vi "Out_S10F1.vi"(8 "error in (no error)":errorcluster, 10 "S10F1":T1, 11 "S10 Message Class in":refnum<class "S10 Message Class.lvclass">) -> (0 "error out":errorcluster, 3 "S10 Message Class out":refnum<class "S10 Message Class.lvclass">)   [LabVIEW 2020, in "SECS Communication.lvlib" / "S10 Message Class.lvclass"]
uses:
  S10 Message Class.lvclass
  S10F1.ctl
  SECS-II Class/Data Message_List.vi
  SECS-II Class/Data Message_Binary.vi
  SECS-II Class/Data Message_ASCII.vi
  SECS-II Class/SECS-II Class.lvclass
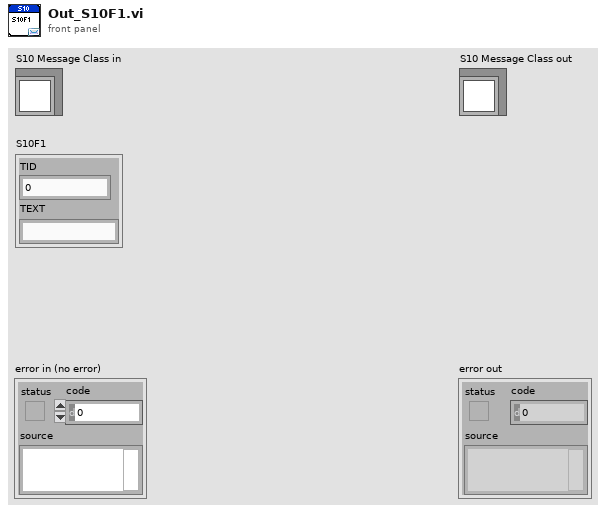
[diagram p1: front panel]
types:
  T1 = typedef "SECS Communication.lvlib/S10 Message Class.lvclass/S10F1.ctl" = cluster{"TID":u8, "TEXT":string}
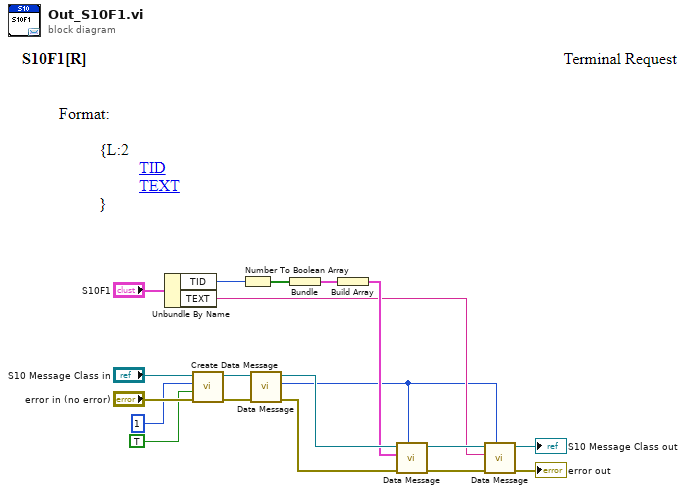
[diagram p0: block diagram]
diagram:
  n1 = Unbundle By Name("S10F1") -> ("TID"=w10:u8, "TEXT"=w4:string)
  n2 = call "Create Data Message.vi"("error in (no error)"="error in (no error)", "W-Bit"=TRUE, "Function"=u8 1, "SECS-II Class in"="S10 Message Class in") -> ("error out"=w18:errorcluster, "SECS-II Class out"=w19:refnum<class "S10 Message Class.lvclass">)  [unwired: 6 in]
  n3 = Number To Boolean Array(number=w10) -> (Boolean array=w9:bool[])
  n4 = call-poly "Data Message.vi"("error in"=w18, "SECS-II Class in"=w19) -> ("error out"=w13:errorcluster, "Index"=w1:i32, "SECS-II Class out"=w12:refnum<class "S10 Message Class.lvclass">)  [unwired: 7 in]
  n5 = Bundle("Boolean array"=w9) -> (w8:cluster{"Boolean array":bool[]})  [unwired: 1 in]
  n6 = Build Array(w8) -> (w7:cluster{"Boolean array":bool[]}[])
  n7 = call-poly "Data Message.vi"("Parent Index"=w1, "error in"=w13, "Data Cluster"=w7, "SECS-II Class in"=w12) -> ("error out"=w5:errorcluster, "SECS-II Class out"=w6:refnum<class "S10 Message Class.lvclass">)  [unwired: 6 in]
  n8 = call-poly "Data Message.vi"("Parent Index"=w1, "error in"=w5, "Data"=w4, "SECS-II Class in"=w6) -> ("error out"=→"error out":errorcluster, "SECS-II Class out"=→"S10 Message Class out":refnum<class "S10 Message Class.lvclass">)  [unwired: 6 in]
